vi "Initialize Sim youBot Platform.vi"(8 "error in":errorcluster, 11 "robot ID":string) -> (0 "error out":errorcluster, 3 "simulated KUKA youBot platform out":refnum<class "NI_Robotics_KUKA youBot Platform_Sim.lvclass">)   [LabVIEW 2017, in "NI_Robotics_KUKA youBot Host.lvlib" / "NI_Robotics_KUKA youBot Platform_Sim.lvclass"]
uses:
  <vilib>/robotics/KUKA youBot/Basic Device/Mobile Platform Sim/NI_Robotics_KUKA youBot Platform_Sim.lvclass
  c:/Program Files (x86)/National Instruments/LabVIEW 2017/vi.lib/robotics/KUKA youBot/Basic Device/Mobile Platform/NI_Robotics_KUKA youBot Platform.lvclass
  <vilib>/robotics/Simulator/Engine/ctl/DeviceID.ctl
  <vilib>/robotics/KUKA youBot/Motor/Wheel Motor Sim/NI_Robotics_KUKA youBot Wheel Motor_Sim.lvclass
  c:/Program Files (x86)/National Instruments/LabVIEW 2017/vi.lib/robotics/KUKA youBot/Motor/Wheel Motor/NI_Robotics_KUKA youBot Wheel Motor.lvclass
  <vilib>/robotics/Simulator/NI_Robotics_Simulator.lvlib
  <vilib>/robotics/KUKA youBot/Basic Device/Mobile Platform/NI_Robotics_KUKA youBot Platform.lvclass
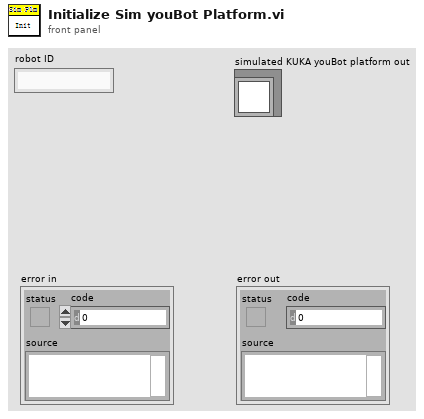
[diagram p1: front panel]
types:
  T1 = typedef "NI_Robotics_Simulator.lvlib/DeviceID.ctl" = cluster{"robot ID":string, "sensor/actuator ID":string}
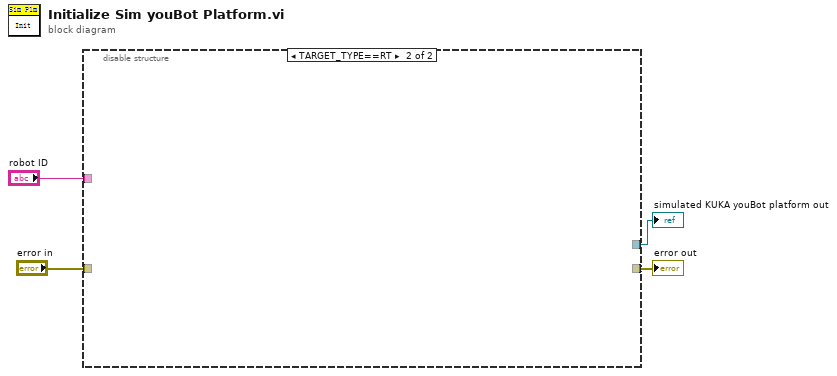
[diagram p0: block diagram]
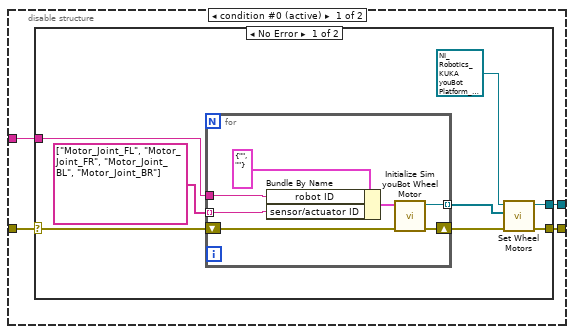
[diagram p2: hidden frame]
diagram:
  n1 = disable-structure shown="TARGET_TYPE==RT" {
    disable-tunnel: "error in" -> [w8 _]
    disable-tunnel: "robot ID" -> [w7 _]
    disable-tunnel: [w6 _] -> w2
    disable-tunnel: [w5 _] -> w1
    frame condition #0 (active) {
      n2 = case shown="No Error" w8 {
        selector: w8 -> [w14 w24]
        tunnel: w7 -> [w15 _]
        tunnel: [w10 w24] -> w6
        tunnel: [w9 _] -> w5
        frame No Error {
          n3 = for {
            tunnel: string[] ["Motor_Joint_FL", "Motor_Joint_FR", "Motor_Joint_BL", "Motor_Joint_BR"] -> [w22] mode=indexing
            shift-right: [w19] -> w11
            shift-left: w14 -> [w20]
            tunnel: w15 -> [w21]
            tunnel: [w17] -> w12 mode=indexing
            n4 = Bundle By Name(cluster=T1 {"robot ID"="", "sensor/actuator ID"=""} ("Device ID"), "robot ID"=w21, "sensor/actuator ID"=w22) -> (w18:T1)
            n5 = call <vilib>:"Initialize Sim youBot Wheel Motor.vi"("error in (no error)"=w20, "device ID"=w18) -> ("error out"=w19:errorcluster, "simulated KUKA youBot wheel motor out"=w17:refnum<class "NI_Robotics_KUKA youBot Wheel Motor_Sim.lvclass">)  [unwired: 8 in]
          }
          n6 = call <vilib>:"Set Wheel Motors.vi"("error in (no error)"=w11, "wheel motors"=w12, "KUKA youBot platform in"=refnum<class "NI_Robotics_KUKA youBot Platform_Sim.lvclass"> refnum ("NI_Robotics_KUKA youBot Host.lvlib:NI_Robotics_KUKA youBot Platform_Sim.lvclass")) -> ("error out"=w10:errorcluster, "KUKA youBot platform out"=w9:refnum<class "NI_Robotics_KUKA youBot Platform_Sim.lvclass">)  [unwired: 7 in]
        }
        frame Error {
        }
      }
    }
    frame condition #1 {
    }
  }
  "error out" <- w2
  "simulated KUKA youBot platform out" <- w1
